vi "COMMAND_SetOrigin.vi"(8 "error in (no error)":errorcluster, 11 "MH100301DMC in":refnum<class "StageMH100301DMC.lvclass">) -> (0 "error out":errorcluster, 3 "MH100301DMC out":refnum<class "StageMH100301DMC.lvclass">)   [LabVIEW 2010, in "StageMH100301DMC.lvclass"]
uses:
  StageMH100301DMC.lvclass
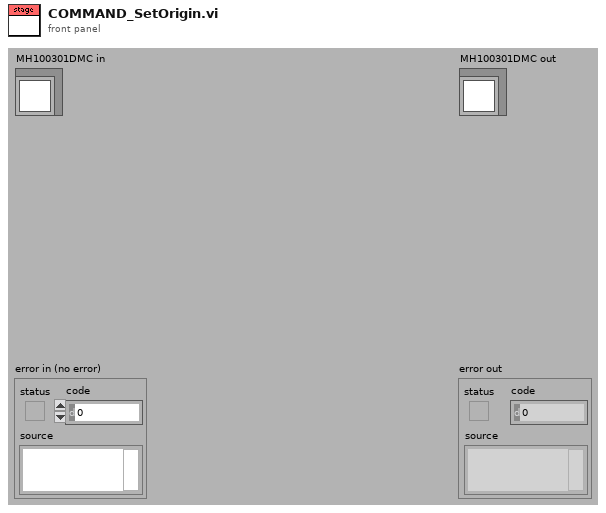
[diagram p1: front panel]
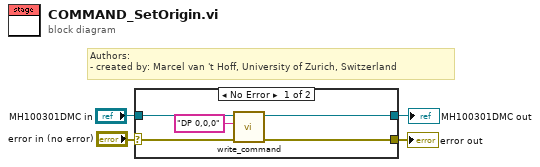
[diagram p0: block diagram]
diagram:
  # "Authors: \n- created by: Marcel van 't Hoff, University of Zurich, Switzerland"
  n1 = case shown="No Error" "error in (no error)" {
    selector: "error in (no error)" -> [w8 w11]
    tunnel: [w7 w11] -> w3
    tunnel: [w6 w10] -> w1
    tunnel: "MH100301DMC in" -> [w9 w10]
    frame No Error {
      n2 = call-dynamic "write_command.vi"("error in (no error)"=w8, "command (without terminating \"\\n\")"="DP 0,0,0" ("command (without terminating \"\\n\")"), "MH100301DMC in"=w9) -> ("error out"=w7:errorcluster, "MH100301DMC out"=w6:refnum<class "StageMH100301DMC.lvclass">)  [unwired: 6 in, 1 out]
    }
    frame Error {
    }
  }
  "error out" <- w3
  "MH100301DMC out" <- w1
